vi "Initialize-client.vi"(8 "error in (no error)":errorcluster, 9 "Client channel":refnum<queue>, 10 "Server channel":refnum<queue>, 11 "Data ref. in":refnum<data-value>) -> (0 "error out":errorcluster, 3 "Data ref.":refnum<data-value>)   [LabVIEW 2013, in "CameraVision.lvlib" / "CV-Main.lvclass"]
uses:
  CV-Main.lvclass
  SA-SLMAPI/Sources/Message.lvclass
  CV-Main.lvclass/CV-Main.ctl
  Client/Sources/CV-Client.lvclass
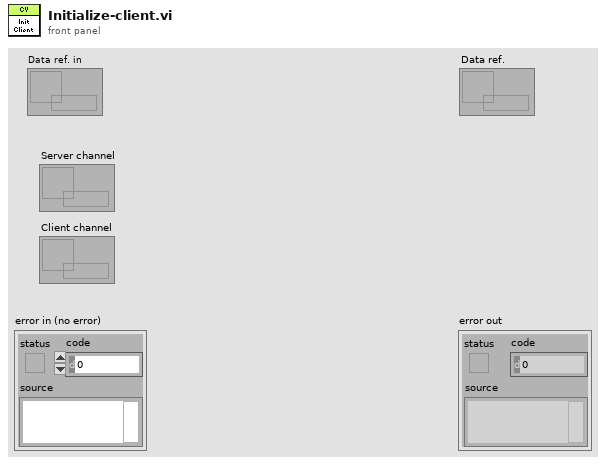
[diagram p1: front panel]
types:
  T1 = typedef "CameraVision.lvlib/CV-Client.lvclass/Object-reference.ctl" = refnum<data-value>
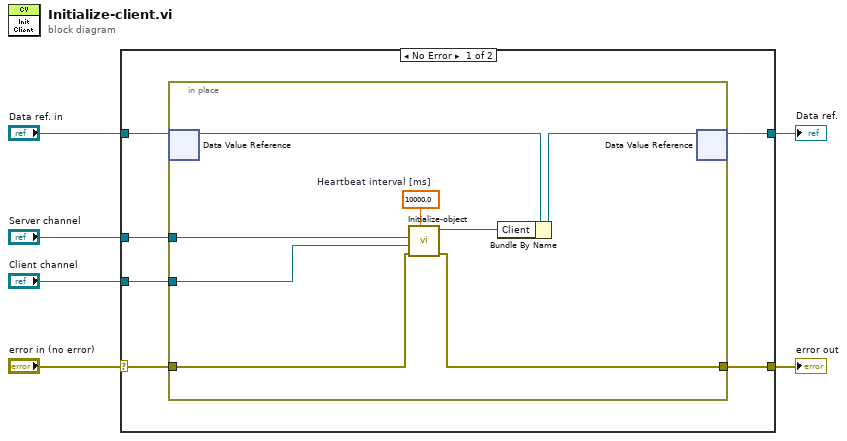
[diagram p0: block diagram]
diagram:
  n1 = case shown="No Error" "error in (no error)" {
    selector: "error in (no error)" -> [w10 w22]
    tunnel: [w9 w22] -> w5
    tunnel: "Data ref. in" -> [w12 w21]
    tunnel: [w11 w21] -> w3
    tunnel: "Client channel" -> [w8 _]
    tunnel: "Server channel" -> [w7 _]
    frame No Error {
      n2 = in-place {
        in-place-border: [w15] -> w9
        in-place-border: w10 -> [w16]
        in-place-border: w8 -> [w14]
        in-place-border: w7 -> [w13]
        w17 = 10000.0  # Heartbeat interval [ms]
        n3 = in-place-dvr #1(w12) -> (w20:refnum<class "CV-Main.lvclass">)  [unwired: 1 out]
        n4 = call "Initialize-object.vi"("Heartbeat interval"=w17, "error in (no error)"=w16, "Client channel"=w14, "Server channel"=w13) -> ("error out"=w15:errorcluster, "Reference out"=w18:T1)  [unwired: 6 in]
        n5 = Bundle By Name(cluster=w20, "Client"=w18) -> (w19:refnum<class "CV-Main.lvclass">)
        n6 = in-place-dvr #1(w19) -> (w11:refnum<data-value>)  [unwired: 1 out]
      }
    }
    frame Error {
    }
  }
  "error out" <- w5
  "Data ref." <- w3
